vi "Periodic Tasks.vi"(8 "error in":errorcluster) -> ()   [LabVIEW 2020]
doc: "This VI runs in parallel to other tasks. It can contain as many user-defined periodic loops as you need. These can carry out PID or other sorts of timed response."
uses:
  Robot Global Data.vi
  <vilib>/Rock Robotics/Network Tables/NT Read Number.vi
panel:
  # "t"
  # "Click here to set max"
  # "Click here to set min"
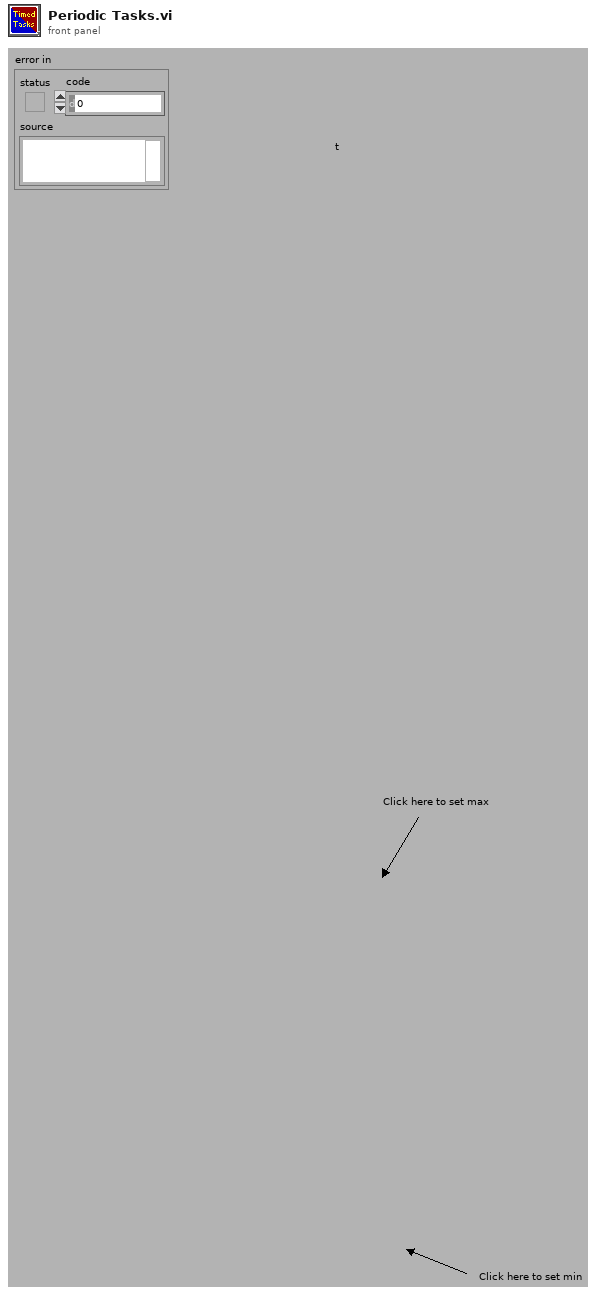
[diagram p1: front panel]
types:
  T1 = typedef "WPI_MotorControlDeviceRef.ctl" = cluster{"DeviceStatus":errorcluster, "Type":T2, "PWM":cluster{"PWM Channel":T3, "DeadBand":T4}, "CAN":cluster{"Device Number":u8, "SetOutput VI Ref":variant, "GetOutput VI Ref":variant, "Enable VI Ref":variant, "Disable VI Ref":variant, "Data":variant}, "Invert":bool, "DIO PWM":cluster{"PWM \"Enable\" Channel":T3, "DIOChannel":T5, "PWM Rate":dbl}}
  T2 = typedef "WPI_MotorControlType.ctl" = enum16{"PWM", "CAN", "DIO PWM"}
  T3 = typedef "FPGA_DIOPWMChannel.ctl" = enum8{"PWM 0", "PWM 1", "PWM 2", "PWM 3", "PWM 4", "PWM 5", "PWM 6", "PWM 7", "PWM 8", "PWM 9", "PWM MXP 0", "PWM MXP 1", "PWM MXP 2", "PWM MXP 3", "PWM MXP 4", "PWM MXP 5", "PWM MXP 6", "PWM MXP 7", "PWM MXP 8", "PWM MXP 9", "Invalid"}
  T4 = typedef "WPI_PWMDeadband.ctl" = cluster{"Name":string, "maxPositivePwm":i32, "minPositivePwm":i32, "centerPwm":i32, "maxNegativePwm":i32, "minNegativePwm":i32, "angularRange":u16}
  T5 = typedef "FPGA_DIOChannel.ctl" = enum8{"DIO 0", "DIO 1", "DIO 2", "DIO 3", "DIO 4", "DIO 5", "DIO 6", "DIO 7", "DIO 8", "DIO 9", "DIO MXP 0", "DIO MXP 1", "DIO MXP 2", "DIO MXP 3", "DIO MXP 4", "DIO MXP 5", "DIO MXP 6", "DIO MXP 7", "DIO MXP 8", "DIO MXP 9", "DIO MXP 10", "DIO MXP 11", "DIO MXP 12", "DIO MXP 13", "DIO MXP 14", "DIO MXP 15", "SPI Port CS1", "SPI Port CS2", "SPI Port CS3", "SPI Port MISO", "SPI Port MOSI", "Invalid"}
  T6 = typedef "WPI_RobotDriveDevRef.ctl" = cluster{"DevStatus":errorcluster, "Motors[]":T1[], "Square Inputs":bool, "Max Output":dbl}
  T7 = typedef "WPI_JoystickDevRef.ctl" = cluster{"Device":T8}
  T8 = typedef "WPI_JoystickDeviceEnum.ctl" = enum16{"USB 0", "USB 1", "USB 2", "USB 3", "USB 4", "USB 5"}
  T9 = cluster{"JoystickDevRef":T7, "RobotDriveDevRef":T6, "Numeric":dbl, "Numeric":dbl, "MotorControlDevRef":T1, "MotorControlDevRef":T1}
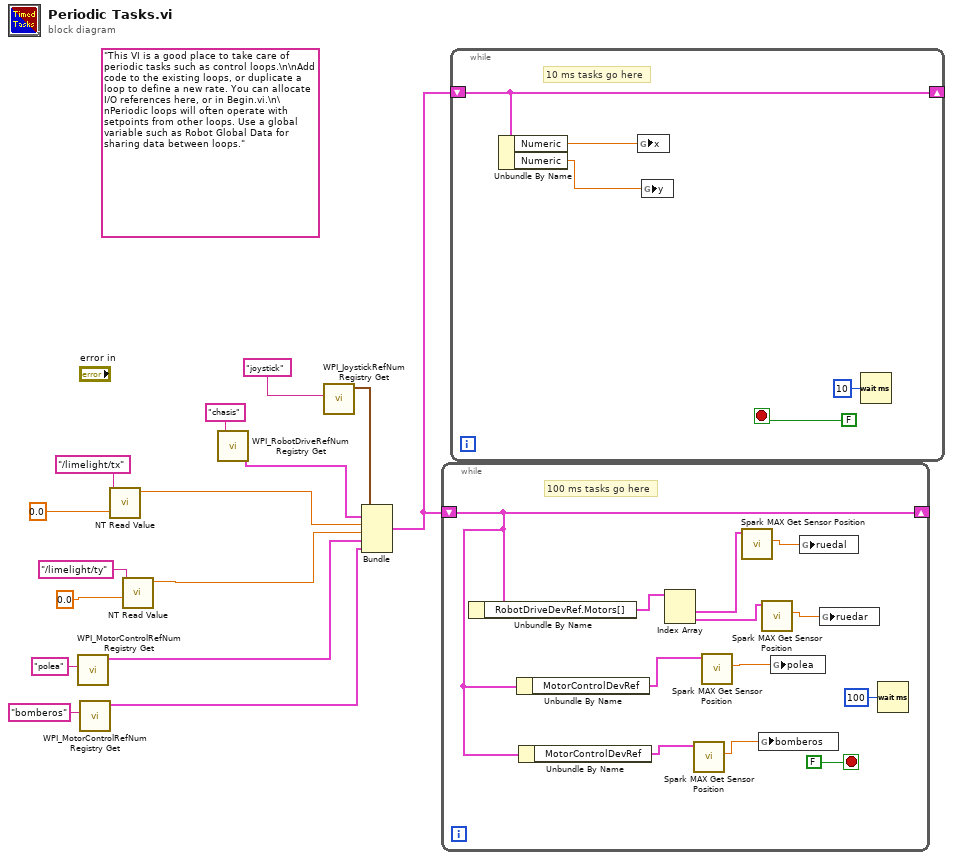
[diagram p0: block diagram]
diagram:
  (unwired) "This VI is a good place to take care of periodic tasks such as control loops.\n\nAdd code to the existing loops, or duplicate a loop to define a new rate. You can allocate I/O references here, or in Begin.vi.\n\nPeriodic loops will often operate with setpoints from other loops. Use a global variable such as Robot Global Data for sharing data between loops."
  n1 = call <vilib>:"WPI_MotorControlRefNum Registry Get.vi"("refnum name"="polea") -> ("MotorControlDevRef"=w4:T1)  [unwired: 9 in, 1 out]
  n2 = call <vilib>:"WPI_MotorControlRefNum Registry Get.vi"("refnum name"="bomberos") -> ("MotorControlDevRef"=w1:T1)  [unwired: 9 in, 1 out]
  n3 = call-poly <vilib>:"NT Read Value.vi"("Default Value"=0.0, "Name"="/limelight/tx") -> ("Numeric"=w6:dbl)  [unwired: 8 in, 1 out]
  n4 = call-poly <vilib>:"NT Read Value.vi"("Default Value"=0.0, "Name"="/limelight/ty") -> ("Numeric"=w5:dbl)  [unwired: 8 in, 1 out]
  n5 = call <vilib>:"WPI_RobotDriveRefNum Registry Get.vi"("refnum name"="chasis") -> ("RobotDriveDevRef"=w12:T6)  [unwired: 1 in, 9 out]
  n6 = call <vilib>:"WPI_JoystickRefNum Registry Get.vi"("refnum name"="joystick") -> ("JoystickDevRef"=w13:T7)  [unwired: 1 in, 9 out]
  n7 = Bundle("JoystickDevRef"=w13, "RobotDriveDevRef"=w12, "Numeric"=w6, "Numeric"=w5, "MotorControlDevRef"=w4, "MotorControlDevRef"=w1) -> (w11:T9)  [unwired: 1 out]
  n8 = while {
    shift-right: [w23] -> _
    shift-left: w11 -> [w23]
    stop <- FALSE stop-if-true
    # "100 ms tasks go here"
    n9 = Unbundle By Name(w23) -> ("RobotDriveDevRef.Motors[]"=w25:T1[])
    n10 = Unbundle By Name(w23) -> ("MotorControlDevRef"=w20:T1)
    n11 = Unbundle By Name(w23) -> ("MotorControlDevRef"=w22:T1)
    n12 = Index Array(array=w25) -> (element #1=w18:T1, element #2=w17:T1)  [unwired: 2 in]
    n13 = call <vilib>:"Spark MAX Get Sensor Position.vi"("MotorControlDevRef in"=w22) -> ("Sensor Position"=w21:dbl)  [unwired: 7 in, 3 out]
    n14 = call <vilib>:"Spark MAX Get Sensor Position.vi"("MotorControlDevRef in"=w20) -> ("Sensor Position"=w19:dbl)  [unwired: 7 in, 3 out]
    n15 = call <vilib>:"Spark MAX Get Sensor Position.vi"("MotorControlDevRef in"=w18) -> ("Sensor Position"=w24:dbl)  [unwired: 7 in, 3 out]
    n16 = global write "Robot Global Data.vi" "bomberos"(w21) -> ()
    n17 = call <vilib>:"Spark MAX Get Sensor Position.vi"("MotorControlDevRef in"=w17) -> ("Sensor Position"=w16:dbl)  [unwired: 7 in, 3 out]
    n18 = global write "Robot Global Data.vi" "polea"(w19) -> ()
    n19 = global write "Robot Global Data.vi" "ruedal"(w24) -> ()
    n20 = global write "Robot Global Data.vi" "ruedar"(w16) -> ()
    n21 = Wait (ms)(milliseconds to wait=u32 100) -> ()  [unwired: 1 out]
  }
  n22 = while {
    shift-right: [w30] -> _
    shift-left: w11 -> [w30]
    stop <- FALSE stop-if-true
    # "10 ms tasks go here"
    n23 = Unbundle By Name(w30) -> ("Numeric"=w29:dbl, "Numeric"=w28:dbl)
    n24 = global write "Robot Global Data.vi" "x"(w29) -> ()
    n25 = global write "Robot Global Data.vi" "y"(w28) -> ()
    n26 = Wait (ms)(milliseconds to wait=u32 10) -> ()  [unwired: 1 out]
  }
